vi "KX-100L_basics.vi"() -> ()   [LabVIEW 2017]
panel:
  in  "INPUT":string
  out "OUTPUT":string
  in  "Action\n [SetVoltage, SetCurrent, OutputOn, OutputOff, GetStatus]":T1(ring)
  out "エラー出力":errorcluster
  in  "エラー入力（エラーなし）":errorcluster
  in  "Device [0 or 1]":i32=2
  in  "VISAリソース名":refnum<visa-resource-name>
  # "In/out for ControllerX"
  # "Choose 1 for UCN polarization exp. March 2022"
  # "Local controls/indicators"
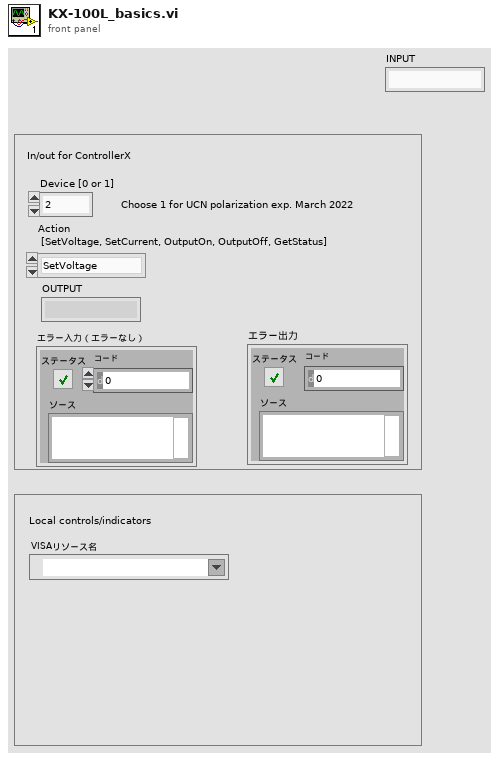
[diagram p1: front panel]
types:
  T1 = enum16{"SetVoltage", "SetCurrent", "OutputOn", "OutputOff", "ReadStatus"}
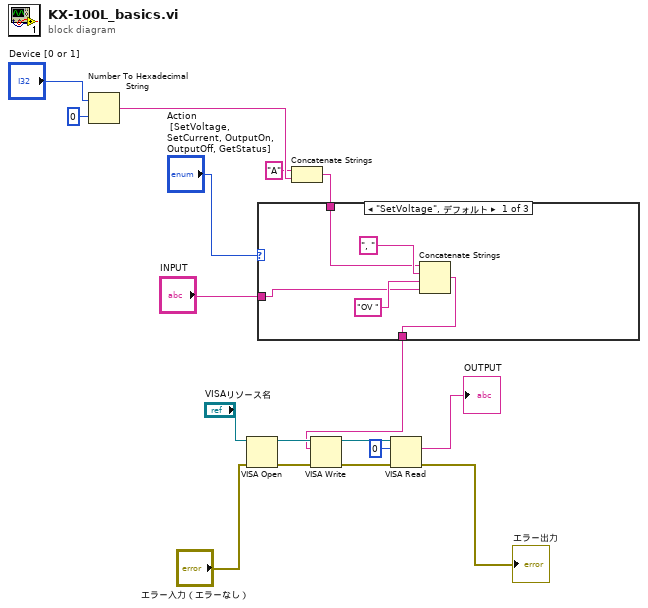
[diagram p0: block diagram]
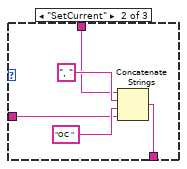
[diagram p2: hidden frame]
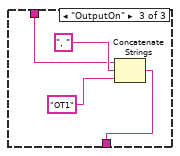
[diagram p3: hidden frame]
diagram:
  n1 = Number To Hexadecimal String(1:i16 0 ("幅（-）"), 2:"Device [0 or 1]") -> (0:w5:string)
  n2 = VISA Open(error in (no error)="エラー入力（エラーなし）", VISA resource name="VISAリソース名") -> (VISA resource name=w15:refnum<visa-resource-name>, error out=w14:errorcluster)  [unwired: 3 in]
  n3 = Concatenate Strings("A" ("文字列"), w5) -> (w2:string)
  n4 = case shown="\"SetVoltage\", デフォルト" "Action\n [SetVoltage, SetCurrent, OutputOn, OutputOff, GetStatus]" {
    tunnel: "INPUT" -> [w19 w26 _]
    tunnel: w2 -> [w20 w24 w28]
    tunnel: [w18 w23 w29] -> w1
    frame "SetVoltage", Default {
      n5 = Concatenate Strings(w20, ", " ("書き込みバッファ"), "OV " ("書き込みバッファ"), w19) -> (w18:string)
    }
    frame "SetCurrent" {
      n6 = Concatenate Strings(w24, ", " ("書き込みバッファ"), "OC " ("書き込みバッファ"), w26) -> (w23:string)
    }
    frame "OutputOn" {
      n7 = Concatenate Strings(w28, ", " ("書き込みバッファ"), "OT1" ("書き込みバッファ")) -> (w29:string)
    }
  }
  n8 = VISA Write(VISA resource name=w15, write buffer=w1, error in (no error)=w14) -> (VISA resource name out=w9:refnum<visa-resource-name>, error out=w8:errorcluster)  [unwired: 1 out]
  n9 = VISA Read(VISA resource name=w9, byte count=u32 0 ("バイトカウント"), error in (no error)=w8) -> (read buffer=→"OUTPUT":string, error out=→"エラー出力":errorcluster)  [unwired: 2 out]
